vi "Write ConfigDir.vi"(8 "error in (no error)":errorcluster, 10 "ConfigDir":path, 11 "HIJ Vision Application in":refnum<class "HIJ Vision Application.lvclass">) -> (0 "error out":errorcluster, 3 "HIJ Vision Application out":refnum<class "HIJ Vision Application.lvclass">)   [LabVIEW 2020, in "HIJ Vision Application.lvlib" / "HIJ Vision Application.lvclass"]
uses:
  HIJ Vision Application.lvclass
  HIJ Vision Application.lvclass/HIJ Vision Application.ctl
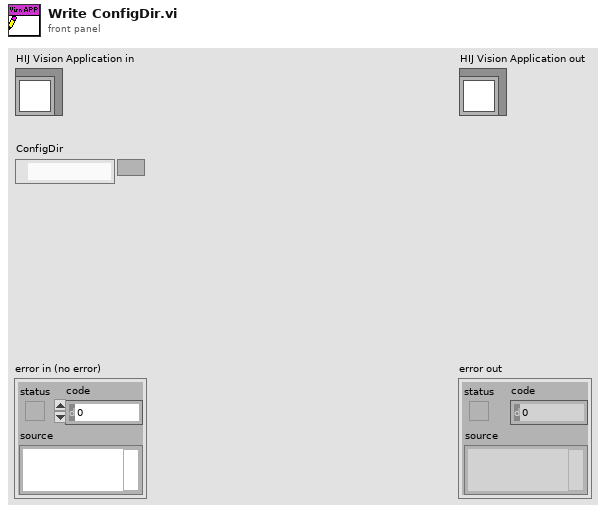
[diagram p1: front panel]
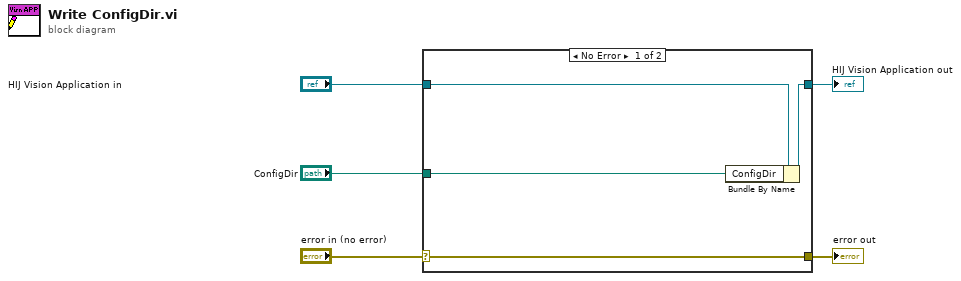
[diagram p0: block diagram]
diagram:
  n1 = case shown="No Error" "error in (no error)" {
    selector: "error in (no error)" -> [w9 w10]
    tunnel: [w9 w10] -> w4
    tunnel: [w7 w11] -> w2
    tunnel: "HIJ Vision Application in" -> [w8 w11]
    tunnel: "ConfigDir" -> [w6 _]
    frame No Error {
      n2 = Bundle By Name(cluster=w8, "ConfigDir"=w6) -> (w7:refnum<class "HIJ Vision Application.lvclass">)
    }
    frame Error {
    }
  }
  "error out" <- w4
  "HIJ Vision Application out" <- w2
